vi "Execute Command.vi"   [LabVIEW 2020, in "SLSC.lvlib"]
doc: "Executes the specified command on one or multiple devices or physical channels."
uses:
  <vilib>/SLSC/SLSC.lvlib
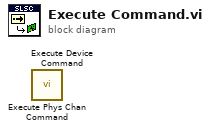
[diagram p0: block diagram]
diagram:
  n1 = call <vilib>:"Execute Phys Chan Command.vi"() -> ()  [unwired: 14 in, 2 out]
  n2 = call <vilib>:"Execute Device Command.vi"() -> ()  [unwired: 14 in, 2 out]
